vi "测试类型2增加一条自动测试记录.vi"(8 "测试结果":string, 9 "最大误差":dbl, 10 "输入通道":i32, 11 "输出通道":i32) -> ()   [LabVIEW 2010]
uses:
  全局量/自动测试结果.vi
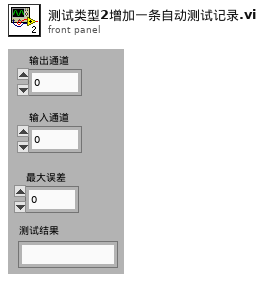
[diagram p1: front panel]
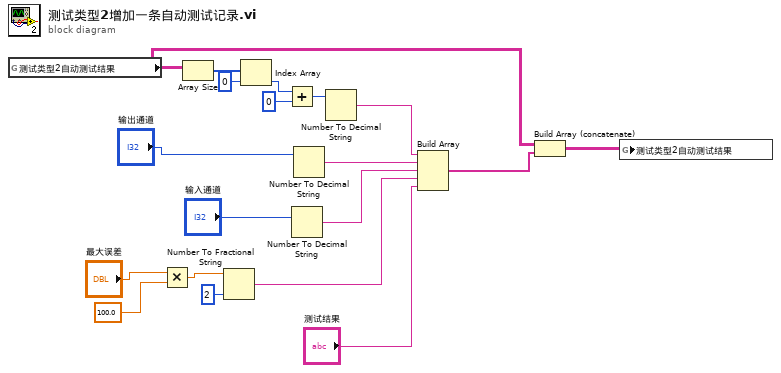
[diagram p0: block diagram]
diagram:
  n1 = global read "自动测试结果.vi" "测试类型2自动测试结果"() -> (w14:string[][])
  n2 = Multiply(x="最大误差", y=100.0) -> (x*y=w7:dbl)
  n3 = Array Size(array=w14) -> (size(s)=w19:i32[])
  n4 = Number To Fractional String(number=w7, precision (6)=i16 2 ("精度(6)")) -> (F-format string=w10:string)  [unwired: 2 in]
  n5 = Index Array(array=w19, index=0 ("索引")) -> (element=w17:i32)
  n6 = Add(x=w17, y=0) -> (x+y=w15:i32)
  n7 = Number To Decimal String(number="输入通道") -> (decimal integer string=w3:string)  [unwired: 1 in]
  n8 = Number To Decimal String(number="输出通道") -> (decimal integer string=w4:string)  [unwired: 1 in]
  n9 = Number To Decimal String(number=w15) -> (decimal integer string=w5:string)  [unwired: 1 in]
  n10 = Build Array(w5, w4, w3, w10, "测试结果") -> (w13:string[])
  n11 = Build Array (concatenate)(w14, w13) -> (w12:string[][])
  n12 = global write "自动测试结果.vi" "测试类型2自动测试结果"(w12) -> ()
